vi "S2DS_Change DC settingss.vi"(2 "Channel names":string[](array[string]), 3 "DC Info list":T1) -> (1 "DC Info list 2":T1)   [LabVIEW 2025]
uses:
  TYPE DEFS/S2DS_DAC info new.ctl
  TYPE DEFS/S2DS_Single DC info.ctl
panel:
  in  "New DC parameters 3":dbl[](array[numeric])
  out "Updated DC parameters 2":dbl[](array[numeric])
  out "Old DC parameters":dbl[](array[numeric])
  in  "EXIT":bool
  out "V":i32
  out "U":i32
  out "Array":string[](array[string])
  in  "V":i32(ring)
  in  "U":u16(ring)
  out "Wait (ms)":i32
  out "Averaging":i32
  in  "select channel to edit":u16(ring) items=["AbyB"]
  in  "Cancel":bool
  in  "OK":bool
  # "Edit data analysis channel info..."
  # "Parameter name"
  # "Old"
  # "Updated"
  # "Enter new"
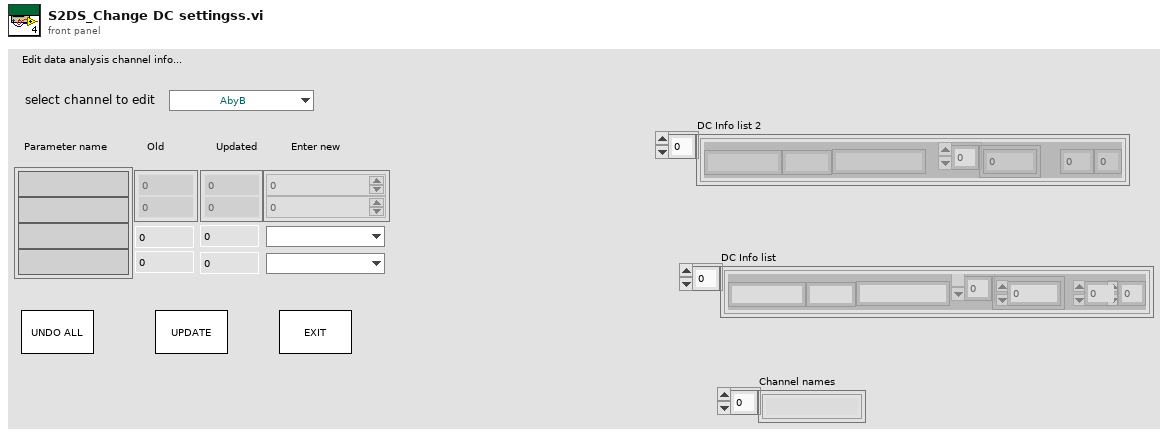
[diagram p1: front panel]
types:
  T1 = typedef "S2DS_DAC info new.ctl" = T2[]
  T2 = typedef "S2DS_Single DC info.ctl" = cluster{"Operation identifier":string, "DC parameters":dbl[], "U":i32, "V":i32, "Name":string, "Unit":string}
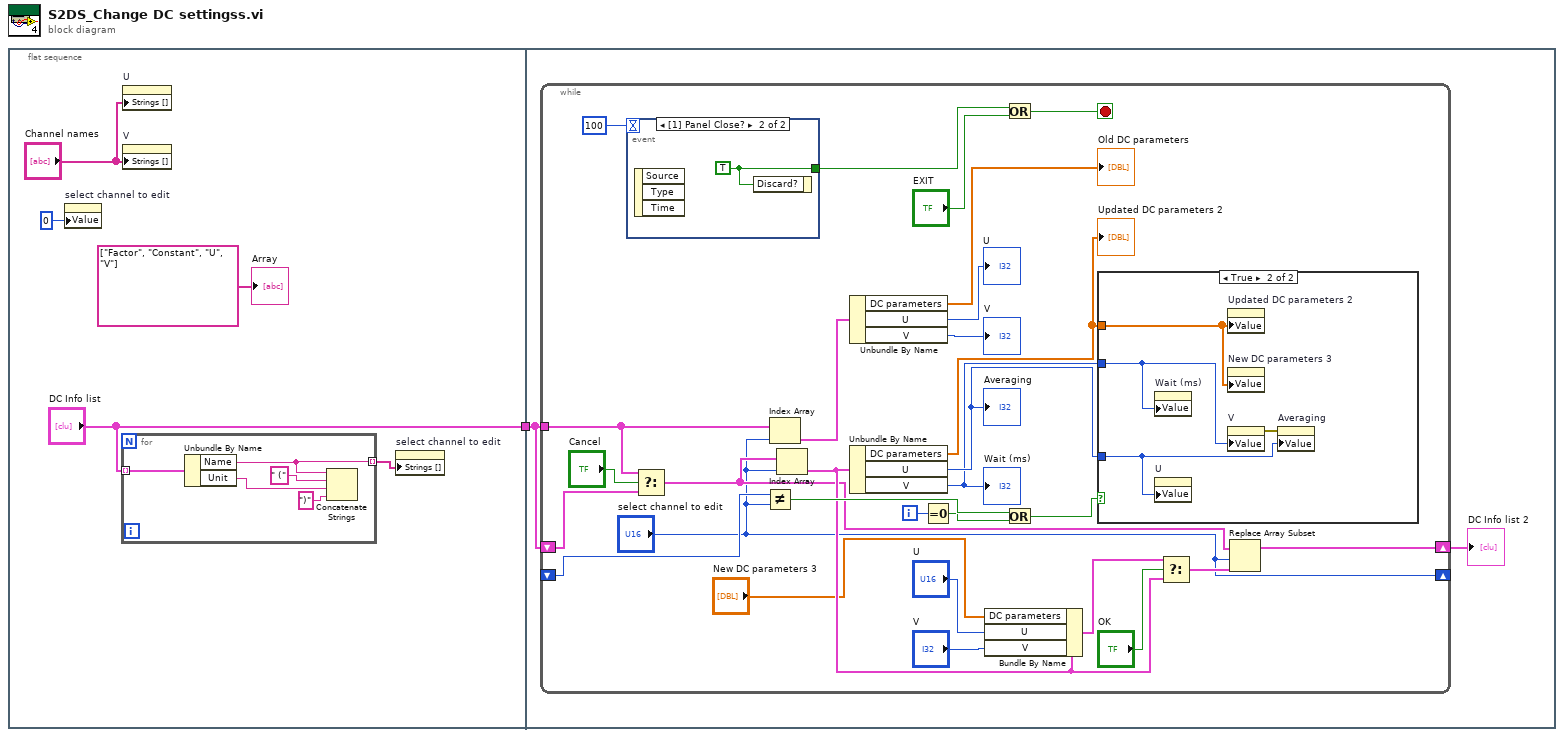
[diagram p0: block diagram]
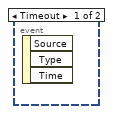
[diagram p2: hidden frame]
diagram:
  n1 = flat-sequence {
    tunnel: ["DC Info list"] -> w1
    tunnel: w1 -> [w13]
    frame #0 {
      n2 = property on="select channel to edit" class="Ring (strict)"("Value"=0) -> ()  [unwired: 2 in, 2 out]
      n3 = for {
        tunnel: "DC Info list" -> [w11] mode=indexing
        tunnel: [w10] -> w4 mode=indexing
        n4 = Unbundle By Name(w11) -> ("Name"=w10:string, "Unit"=w8:string)
        n5 = Concatenate Strings(w10, " (" ("string"), w8, ")" ("string")) -> ()  [unwired: 1 out]
      }
      n6 = property on="U" class="Ring (strict)"("Strings []"="Channel names") -> ()  [unwired: 2 in, 2 out]
      n7 = property on="V" class="Ring (strict)"("Strings []"="Channel names") -> ()  [unwired: 2 in, 2 out]
      n8 = property on="select channel to edit" class="Ring (strict)"("Strings []"=w4) -> ()  [unwired: 2 in, 2 out]
      "Array" <- string[] ["Factor", "Constant", "U", "V"] ("Array")
    }
    frame #1 {
      n9 = while {
        shift-right: [w29] -> w12
        shift-left: w13 -> [w26]
        shift-right: ["select channel to edit"] -> _
        shift-left: _ -> [w42]
        tunnel: w13 -> [w24]
        i -> [w41]
        stop <- w17 stop-if-true
        n10 = event shown="[1] Panel Close?" {
          selector: _ -> [_ _]
          dyn-events: _ -> [_ _]
          timeout: 100 -> [_ _]
          tunnel: [_ w43] -> w18
          event Timeout {
            n11 = event-data() -> ()  [unwired: 1 in, 3 out]
          }
          event Panel Close? {
            w43 = TRUE ("Discard?")
            n12 = event-data() -> ()  [unwired: 1 in, 3 out]
            n13 = event-data("Discard?"=w43) -> ()  [unwired: 1 in, 1 out]
          }
        }
        n14 = Select(t=w24, s="Cancel", f=w26) -> (s? t:f=w25:T1)
        n15 = Not Equal?(x=w42, y="select channel to edit") -> (x != y?=w40:bool)
        n16 = Index Array(array=w24, index="select channel to edit") -> (element=w22:T2)
        n17 = Index Array(array=w25, index="select channel to edit") -> (element=w31:T2)
        n18 = Unbundle By Name(w22) -> ("DC parameters"=→"Old DC parameters":dbl[], "U"=→"U":i32, "V"=→"V":i32)
        n19 = Unbundle By Name(w31) -> ("DC parameters"=w15:dbl[], "U"=w37:i32, "V"=w36:i32)
        "Averaging" <- w37
        "Wait (ms)" <- w36
        "Updated DC parameters 2" <- w15
        n20 = Equal To 0?(x=w41) -> (x = 0?=w39:bool)
        n21 = Bundle By Name(cluster=w31, "DC parameters"="New DC parameters 3", "U"="U", "V"="V") -> (w32:T2)
        n22 = Or(x=w18, y="EXIT") -> (x .or. y?=w17:bool)
        n23 = Or(x=w40, y=w39) -> (x .or. y?=w38:bool)
        n24 = case shown="True" w38 {
          tunnel: w37 -> [_ w47]
          tunnel: w36 -> [_ w45]
          tunnel: w15 -> [_ w44]
          frame False {
          }
          frame True {
            n25 = property on="Wait (ms)" class="DigNum (strict)"("Value"=w45) -> ()  [unwired: 2 in, 2 out]
            n26 = property on="U" class="Ring (strict)"("Value"=w47) -> ()  [unwired: 2 in, 2 out]
            n27 = property on="Updated DC parameters 2" class="Arr (strict)"("Value"=w44) -> ()  [unwired: 2 in, 2 out]
            n28 = property on="New DC parameters 3" class="Arr (strict)"("Value"=w44) -> ()  [unwired: 2 in, 2 out]
            n29 = property on="V" class="Ring (strict)"("Value"=w45) -> (error out=w46:errorcluster)  [unwired: 2 in, 1 out]
            n30 = property on="Averaging" class="DigNum (strict)"(error in=w46, "Value"=w47) -> ()  [unwired: 1 in, 2 out]
          }
        }
        n31 = Select(t=w32, s="OK", f=w31) -> (s? t:f=w30:T2)
        n32 = Replace Array Subset(array=w25, new element=w30, index="select channel to edit") -> (w29:T1)
      }
      "DC Info list 2" <- w12
    }
  }
